vi "SpeedUp.vi"(8 "error in (no error)":errorcluster, 9 "speed multiplier":dbl, 10 "Duration":dbl, 11 "Snake in":refnum<class "Snake.lvclass">) -> (0 "error out":errorcluster, 3 "Snake out":refnum<class "Snake.lvclass">)   [LabVIEW 2019, in "RT_Game.lvlib" / "Snake.lvclass"]
uses:
  Snake.lvclass
  Snake.lvclass/Snake.ctl
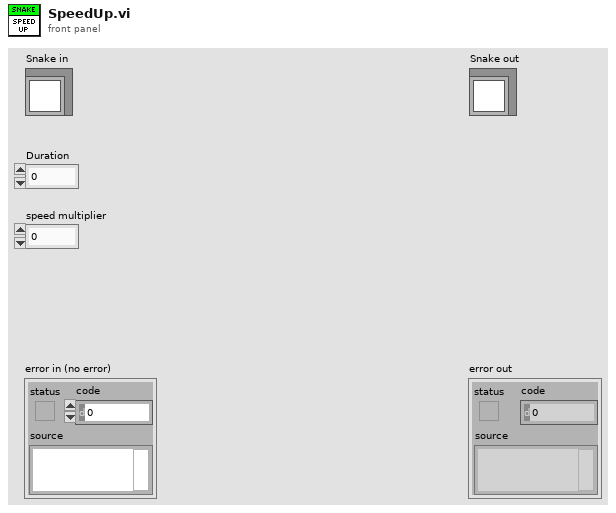
[diagram p1: front panel]
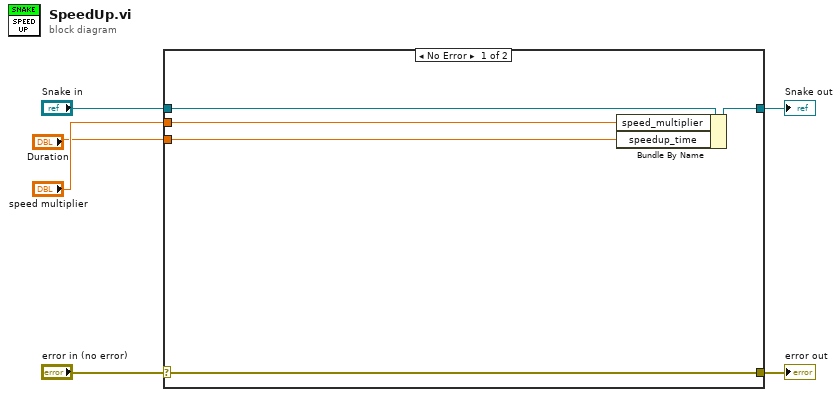
[diagram p0: block diagram]
diagram:
  n1 = case shown="No Error" "error in (no error)" {
    selector: "error in (no error)" -> [w10 w13]
    tunnel: [w10 w13] -> w5
    tunnel: [w9 w12] -> w3
    tunnel: "Snake in" -> [w11 w12]
    tunnel: "speed multiplier" -> [w8 _]
    tunnel: "Duration" -> [w7 _]
    frame No Error {
      n2 = Bundle By Name(cluster=w11, "speed_multiplier"=w8, "speedup_time"=w7) -> (w9:refnum<class "Snake.lvclass">)
    }
    frame Error {
    }
  }
  "error out" <- w5
  "Snake out" <- w3
